vi "Check Register Data Store.vi"(8 "error in (no error)":errorcluster, 10 "register name":string, 11 "register data store in":T1) -> (0 "error IO":errorcluster, 1 "Found":bool, 2 "register offset":u32, 3 "register data store out":T1)   [LabVIEW 2018, in "Scalar IO Operations.lvlib"]
uses:
  Scalar IO Operations.lvlib
  TypeDefs/Register Data Store.ctl
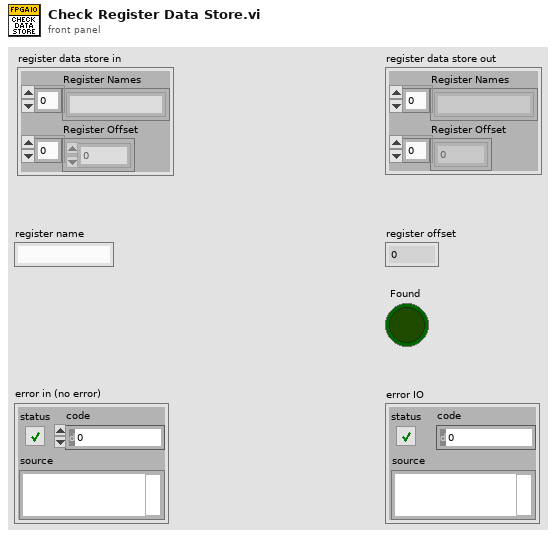
[diagram p1: front panel]
types:
  T1 = typedef "Scalar IO Operations.lvlib/Register Data Store.ctl" = cluster{"Register Names":string[], "Register Offset":u32[]}
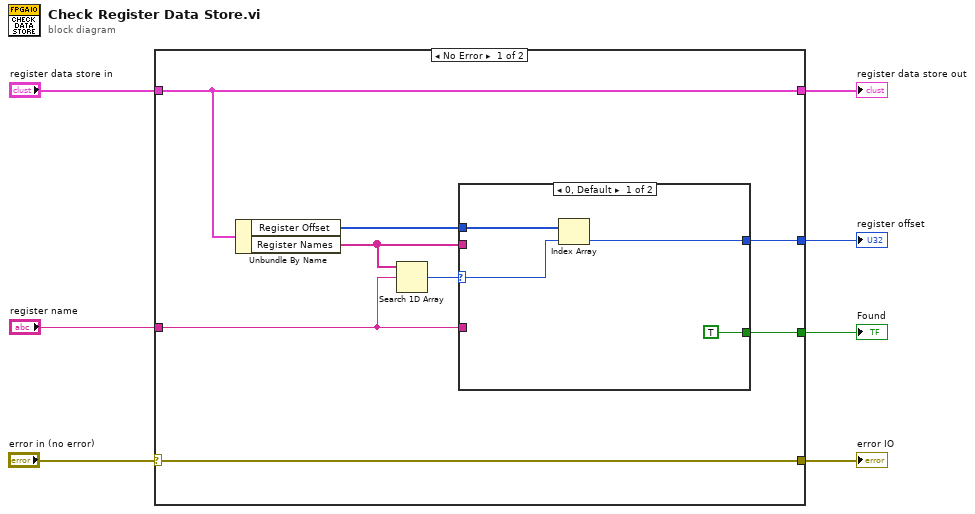
[diagram p0: block diagram]
diagram:
  n1 = case shown="No Error" "error in (no error)" {
    selector: "error in (no error)" -> [w8 w21]
    tunnel: "register name" -> [w15 _]
    tunnel: "register data store in" -> [w9 w20]
    tunnel: [w11 _] -> w5
    tunnel: [w10 _] -> w4
    tunnel: [w9 w20] -> w2
    tunnel: [w8 w21] -> w1
    frame No Error {
      n2 = Unbundle By Name(w9) -> ("Register Offset"=w14:u32[], "Register Names"=w13:string[])
      n3 = Search 1D Array(1D array=w13, element=w15) -> (index of element=w12:i32)  [unwired: 1 in]
      n4 = case shown="0, Default" w12 {
        selector: w12 -> [w18 _]
        tunnel: w13 -> [_ _]
        tunnel: w14 -> [w19 _]
        tunnel: [w17 _] -> w11
        tunnel: w15 -> [_ _]
        tunnel: [TRUE _] -> w10
        frame 0, Default {
          n5 = Index Array(array=w19, index=w18) -> (element=w17:u32)
        }
        frame -1 {
        }
      }
    }
    frame Error {
    }
  }
  "register offset" <- w5
  "register data store out" <- w2
  "Found" <- w4
  "error IO" <- w1
